vi "Tool_Unicode Update Ring Control.vi"(5 "Interpret as Unicode (T)":bool=TRUE, 6 "error in (no error)":errorcluster, 7 "Caption":string, 8 "Strings":string[](array[string]), 9 "Ring Control Ref":refnum<vi>) -> (0 "error out":errorcluster)   [LabVIEW 2020]
panel:
  out "Ring Control Ref":refnum<vi>
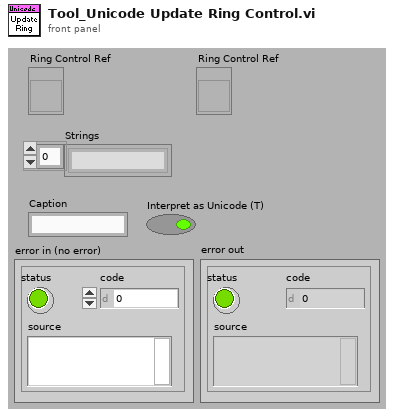
[diagram p1: front panel]
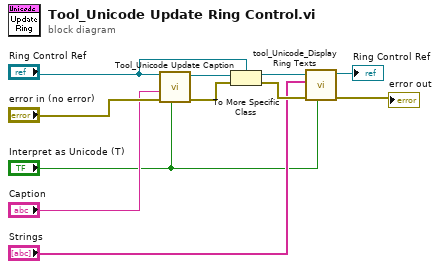
[diagram p0: block diagram]
diagram:
  n1 = call "Tool_Unicode Update Caption.vi"("Interpret as Unicode (T)"="Interpret as Unicode (T)", "error in (no error)"="error in (no error)", "Caption"="Caption", "Control Reference"="Ring Control Ref") -> ("error out"=w8:errorcluster, "Control Reference"=w9:refnum<vi>)  [unwired: 4 in]
  n2 = To More Specific Class(target class="Ring Control Ref", reference=w9, error in=w8) -> (specific class reference=w1:refnum<vi>, error out=w6:errorcluster)
  n3 = call "tool_Unicode_Display Ring Texts.vi"("Interpret as Unicode (T)"="Interpret as Unicode (T)", "error in"=w6, "Ring Texts"="Strings", "Ring Control Ref"=w1) -> ("error out"=→"error out":errorcluster, "Ring Control Ref"=→"Ring Control Ref":refnum<vi>)  [unwired: 4 in]
